vi "Pre Launch Init.vi"(11 "WebSocket Client in":refnum<class "WebSocket Client.lvclass">) -> (0 "error out":errorcluster, 3 "WebSocket Client out":refnum<class "WebSocket Client.lvclass">)   [LabVIEW 2017, in "WebSocket Client.lvlib" / "WebSocket Client.lvclass"]
doc: "(<B>Filename</B>: Actor Framework.lvlib:Actor.lvclass:Pre Launch Init.vi)\n\nDefines behavior that occurs after the Launch Nested Actor method is invoked but before the actor's Actor Core method begins running.\n\nBy default, this method does nothing. A descendant class may override it to define behavior."
uses:
  WebSocket Client.lvclass
  WebSocket Client.lvclass/WebSocket Client.ctl
  Framework/Actor wHelper/Actor wHelper.lvclass
  <vilib>/MediaMongrels Ltd/WebSockets/Sockets/VISA TCP Socket/VISA TCP.lvclass
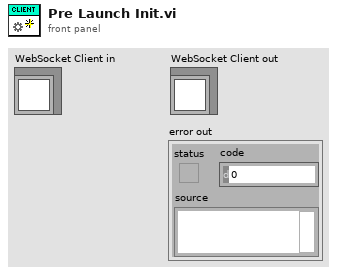
[diagram p1: front panel]
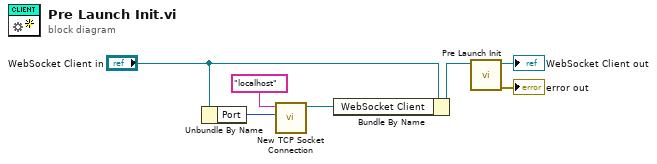
[diagram p0: block diagram]
diagram:
  n1 = Unbundle By Name("WebSocket Client in") -> ("Port"=w2:u16)
  n2 = call <vilib>:"New TCP Socket Connection.vi"("Port"=w2, "Hostname / IP"="localhost" ("format string")) -> ("VISA TCP out"=w1:refnum<class "VISA TCP.lvclass">)  [unwired: 8 in, 1 out]
  n3 = Bundle By Name(cluster="WebSocket Client in", "WebSocket Client"=w1) -> (w4:refnum<class "WebSocket Client.lvclass">)
  n4 = call-parent "Pre Launch Init.vi"("Actor wHelper in"=w4) -> ("error out"=→"error out":errorcluster, "Actor wHelper out"=→"WebSocket Client out":refnum<class "WebSocket Client.lvclass">)  [unwired: 9 in]
